vi "Log Data.vi"(8 "error in (no error)":errorcluster, 10 "Data Queue":T1, 11 "Logging Configuration":T2) -> (0 "error out":errorcluster)   [LabVIEW 2018, in "Logging.lvlib"]
doc: "This VI uses the TDMS Write function to write data to a TDMS file."
uses:
  Logging.lvlib
  Logging Configuration.ctl
  <vilib>/addons/database/Connection.llb/Conn ObjectReference.ctl
  Controls/Data Queue.ctl
  Controls/Acquired Data.ctl
  <vilib>/addons/database/NI_Database_API.lvlib
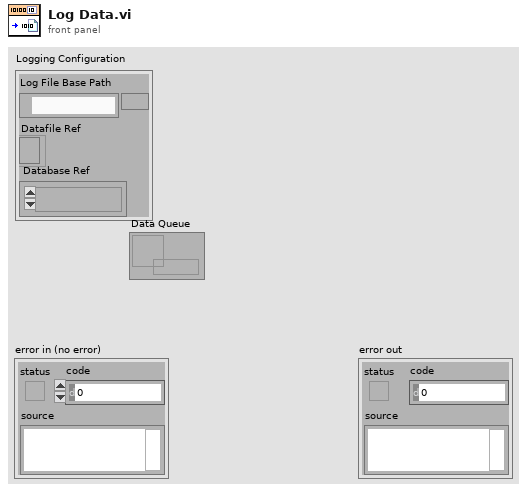
[diagram p1: front panel]
types:
  T1 = typedef "Data Queue.ctl" = refnum<queue>
  T2 = typedef "Logging.lvlib/Logging Configuration.ctl" = cluster{"Log File Base Path":path, "Datafile Ref":refnum<file>, "Database Ref":T3}
  T3 = typedef "NI_Database_API.lvlib/Conn ObjectReference.ctl" = refnum<k1>
  T4 = typedef "Acquired Data.ctl" = cluster{"offset":dbl, "time":string}
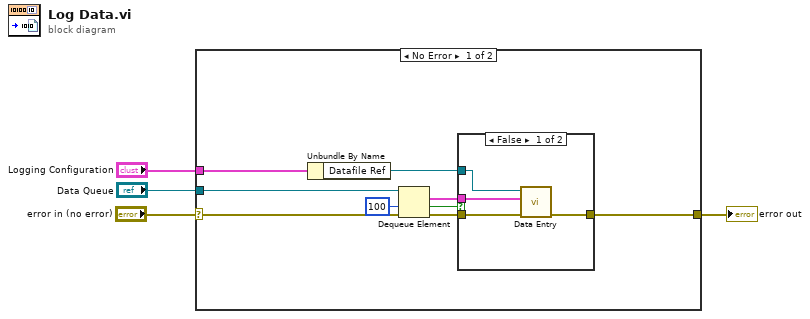
[diagram p0: block diagram]
diagram:
  n1 = case shown="No Error" "error in (no error)" {
    selector: "error in (no error)" -> [w13 w19]
    tunnel: "Logging Configuration" -> [w11 _]
    tunnel: "Data Queue" -> [w12 _]
    tunnel: [w7 w19] -> w3
    frame No Error {
      n2 = Unbundle By Name(w11) -> ("Datafile Ref"=w10:refnum<file>)
      n3 = Dequeue Element(queue=w12, timeout in ms (-1)=100, error in (no error)=w13) -> (element=w9:T4, timed out?=w5:bool, error out=w8:errorcluster)  [unwired: 1 out]
      n4 = case shown="False" w5 {
        tunnel: w10 -> [w17 _]
        tunnel: w9 -> [w16 _]
        tunnel: w8 -> [w15 w18]
        tunnel: [w14 w18] -> w7
        frame False {
          n5 = call "Data Entry.vi"("error in (no error)"=w15, "Data"=w16, "Byte Stream File in"=w17) -> ("error out"=w14:errorcluster)  [unwired: 7 in, 1 out]
        }
        frame True {
        }
      }
    }
    frame Error {
    }
  }
  "error out" <- w3
